vi "Extract BCD Parameter.vi"(8 "Signed?":bool, 9 "numberofBits":i32=19, 10 "startBit":i32=10, 11 "Word":bool[](array[boolean])=[FALSE, FALSE, FALSE, FALSE, FALSE, FALSE, FALSE, FALSE, FALSE, FALSE, FALSE, TRUE, TRUE, FALSE, FALSE, FALSE, FALSE, TRUE, TRUE, TRUE, TRUE, FALSE, TRUE, FALSE, TRUE, FALSE, FALSE, TRUE, FALSE, TRUE, TRUE, FALSE]) -> (3 "BCD Parameter":dbl=25786.0)   [LabVIEW 2019]
doc: "This VI decodes a BCD (signed or not) parameter.\nWhen it's a BCD signed parameter, it's considered negative when SSM bits are 11. For any other combination, we consider it to be positive."
panel:
  # "LSB"
  # "MSB"
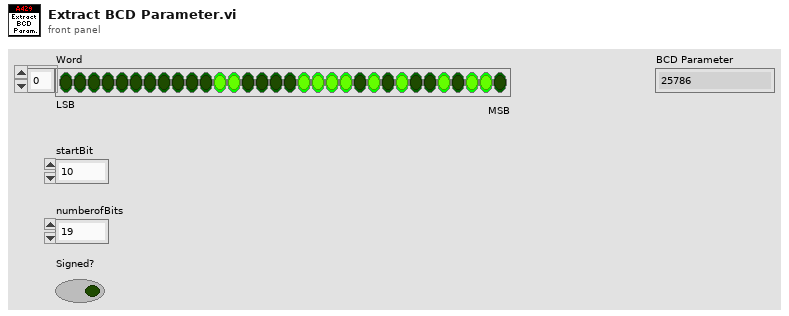
[diagram p1: front panel]
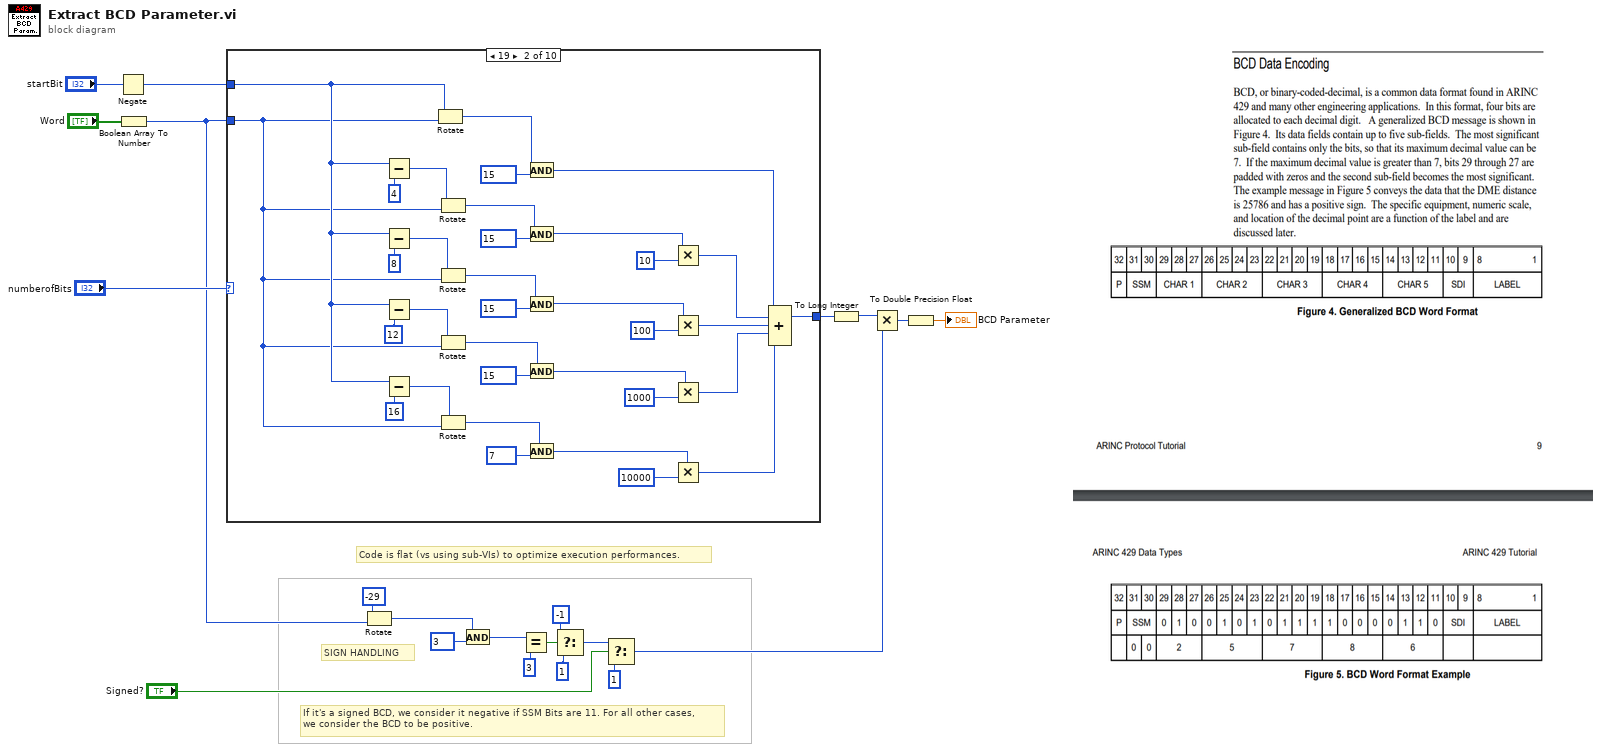
[diagram p0: block diagram]
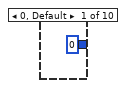
[diagram p2: hidden frame]
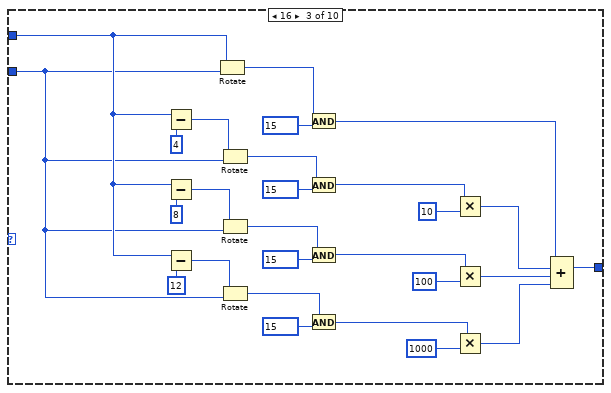
[diagram p3: hidden frame]
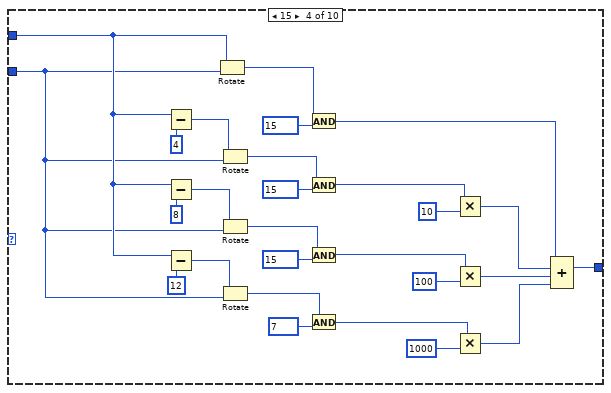
[diagram p4: hidden frame]
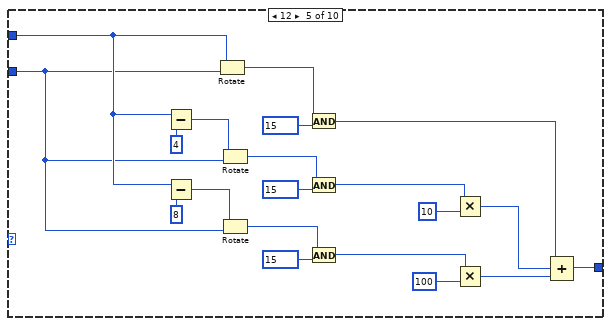
[diagram p5: hidden frame]
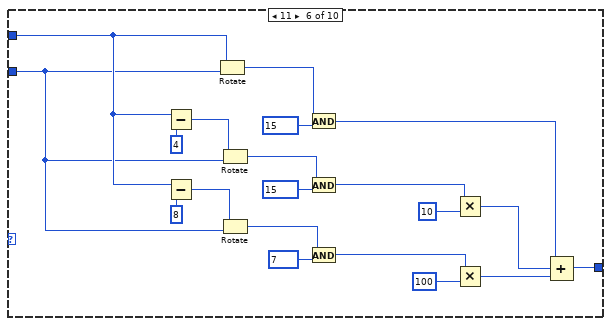
[diagram p6: hidden frame]
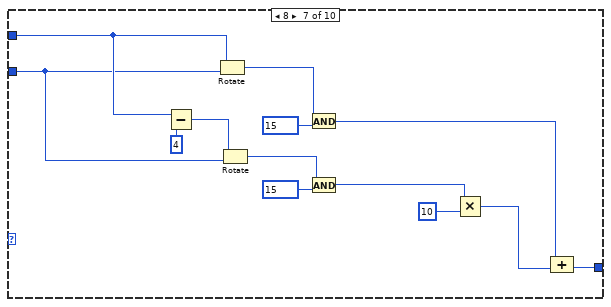
[diagram p7: hidden frame]
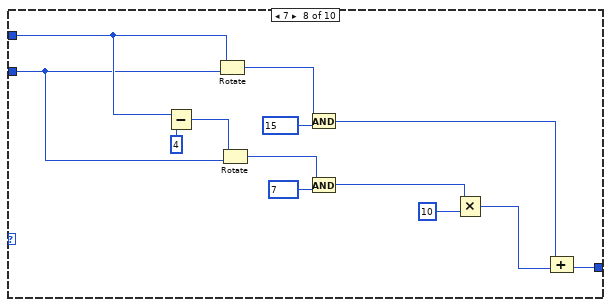
[diagram p8: hidden frame]
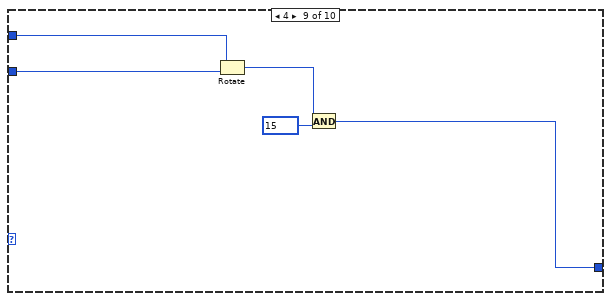
[diagram p9: hidden frame]
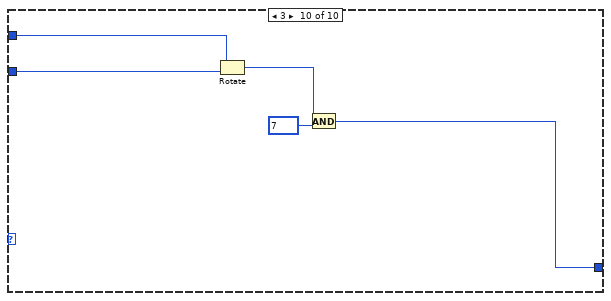
[diagram p10: hidden frame]
diagram:
  # "Code is flat (vs using sub-VIs) to optimize execution performances."
  # "If it's a signed BCD, we consider it negative if SSM Bits are 11. For all other cases,\nwe consider the BCD to be positive."
  # "SIGN HANDLING"
  n1 = Negate(x="startBit") -> (-x=w8:i32)
  n2 = Boolean Array To Number(Boolean array="Word") -> (number=w3:u32)
  n3 = case shown="19" "numberofBits" {
    tunnel: w8 -> [_ w25 w59 w86 w113 w133 w153 w166 w179 w184]
    tunnel: w3 -> [_ w24 w58 w85 w112 w132 w152 w165 w178 w183]
    tunnel: [u32 0 w23 w57 w84 w111 w131 w151 w164 w177 w182] -> w9
    frame 0, Default {
    }
    frame 19 {
      n4 = Subtract(x=w25, y=4) -> (x-y=w48:i32)
      n5 = Subtract(x=w25, y=8) -> (x-y=w42:i32)
      n6 = Subtract(x=w25, y=12) -> (x-y=w26:i32)
      n7 = Subtract(x=w25, y=16) -> (x-y=w27:i32)
      n8 = Rotate(1:w24, 2:w25) -> (0:w56:u32)
      n9 = Rotate(1:w24, 2:w48) -> (0:w52:u32)
      n10 = Rotate(1:w24, 2:w42) -> (0:w46:u32)
      n11 = Rotate(1:w24, 2:w26) -> (0:w40:u32)
      n12 = Rotate(1:w24, 2:w27) -> (0:w34:u32)
      n13 = And(x=w56, y=u32 15) -> (x .and. y?=w53:u32)
      n14 = And(x=w52, y=u32 15) -> (x .and. y?=w50:u32)
      n15 = And(x=w46, y=u32 15) -> (x .and. y?=w44:u32)
      n16 = And(x=w40, y=u32 15) -> (x .and. y?=w38:u32)
      n17 = And(x=w34, y=u32 7) -> (x .and. y?=w32:u32)
      n18 = Multiply(x=w50, y=u32 10) -> (x*y=w37:u32)
      n19 = Multiply(x=w44, y=u32 100) -> (x*y=w36:u32)
      n20 = Multiply(x=w38, y=u32 1000) -> (x*y=w31:u32)
      n21 = Multiply(x=w32, y=u32 10000) -> (x*y=w30:u32)
      n22 = Compound Arithmetic op=ADD(w53, w37, w36, w31, w30) -> (w23:u32)
    }
    frame 16 {
      n23 = Subtract(x=w59, y=4) -> (x-y=w75:i32)
      n24 = Subtract(x=w59, y=8) -> (x-y=w69:i32)
      n25 = Subtract(x=w59, y=12) -> (x-y=w60:i32)
      n26 = Rotate(1:w58, 2:w59) -> (0:w83:u32)
      n27 = Rotate(1:w58, 2:w75) -> (0:w79:u32)
      n28 = Rotate(1:w58, 2:w69) -> (0:w73:u32)
      n29 = Rotate(1:w58, 2:w60) -> (0:w67:u32)
      n30 = And(x=w83, y=u32 15) -> (x .and. y?=w80:u32)
      n31 = And(x=w79, y=u32 15) -> (x .and. y?=w77:u32)
      n32 = And(x=w73, y=u32 15) -> (x .and. y?=w71:u32)
      n33 = And(x=w67, y=u32 15) -> (x .and. y?=w65:u32)
      n34 = Multiply(x=w77, y=u32 10) -> (x*y=w64:u32)
      n35 = Multiply(x=w71, y=u32 100) -> (x*y=w63:u32)
      n36 = Multiply(x=w65, y=u32 1000) -> (x*y=w62:u32)
      n37 = Compound Arithmetic op=ADD(w80, w64, w63, w62) -> (w57:u32)
    }
    frame 15 {
      n38 = Subtract(x=w86, y=4) -> (x-y=w102:i32)
      n39 = Subtract(x=w86, y=8) -> (x-y=w96:i32)
      n40 = Subtract(x=w86, y=12) -> (x-y=w87:i32)
      n41 = Rotate(1:w85, 2:w86) -> (0:w110:u32)
      n42 = Rotate(1:w85, 2:w102) -> (0:w106:u32)
      n43 = Rotate(1:w85, 2:w96) -> (0:w100:u32)
      n44 = Rotate(1:w85, 2:w87) -> (0:w94:u32)
      n45 = And(x=w110, y=u32 15) -> (x .and. y?=w107:u32)
      n46 = And(x=w106, y=u32 15) -> (x .and. y?=w104:u32)
      n47 = And(x=w100, y=u32 15) -> (x .and. y?=w98:u32)
      n48 = And(x=w94, y=u32 7) -> (x .and. y?=w92:u32)
      n49 = Multiply(x=w104, y=u32 10) -> (x*y=w91:u32)
      n50 = Multiply(x=w98, y=u32 100) -> (x*y=w90:u32)
      n51 = Multiply(x=w92, y=u32 1000) -> (x*y=w89:u32)
      n52 = Compound Arithmetic op=ADD(w107, w91, w90, w89) -> (w84:u32)
    }
    frame 12 {
      n53 = Subtract(x=w113, y=4) -> (x-y=w122:i32)
      n54 = Subtract(x=w113, y=8) -> (x-y=w116:i32)
      n55 = Rotate(1:w112, 2:w113) -> (0:w130:u32)
      n56 = Rotate(1:w112, 2:w122) -> (0:w126:u32)
      n57 = Rotate(1:w112, 2:w116) -> (0:w120:u32)
      n58 = And(x=w130, y=u32 15) -> (x .and. y?=w127:u32)
      n59 = And(x=w126, y=u32 15) -> (x .and. y?=w124:u32)
      n60 = And(x=w120, y=u32 15) -> (x .and. y?=w118:u32)
      n61 = Multiply(x=w124, y=u32 10) -> (x*y=w115:u32)
      n62 = Multiply(x=w118, y=u32 100) -> (x*y=w114:u32)
      n63 = Compound Arithmetic op=ADD(w127, w115, w114) -> (w111:u32)
    }
    frame 11 {
      n64 = Subtract(x=w133, y=4) -> (x-y=w142:i32)
      n65 = Subtract(x=w133, y=8) -> (x-y=w136:i32)
      n66 = Rotate(1:w132, 2:w133) -> (0:w150:u32)
      n67 = Rotate(1:w132, 2:w142) -> (0:w146:u32)
      n68 = Rotate(1:w132, 2:w136) -> (0:w140:u32)
      n69 = And(x=w150, y=u32 15) -> (x .and. y?=w147:u32)
      n70 = And(x=w146, y=u32 15) -> (x .and. y?=w144:u32)
      n71 = And(x=w140, y=u32 7) -> (x .and. y?=w138:u32)
      n72 = Multiply(x=w144, y=u32 10) -> (x*y=w135:u32)
      n73 = Multiply(x=w138, y=u32 100) -> (x*y=w134:u32)
      n74 = Compound Arithmetic op=ADD(w147, w135, w134) -> (w131:u32)
    }
    frame 8 {
      n75 = Subtract(x=w153, y=4) -> (x-y=w155:i32)
      n76 = Rotate(1:w152, 2:w153) -> (0:w163:u32)
      n77 = Rotate(1:w152, 2:w155) -> (0:w159:u32)
      n78 = And(x=w163, y=u32 15) -> (x .and. y?=w160:u32)
      n79 = And(x=w159, y=u32 15) -> (x .and. y?=w157:u32)
      n80 = Multiply(x=w157, y=u32 10) -> (x*y=w154:u32)
      n81 = Compound Arithmetic op=ADD(w160, w154) -> (w151:u32)
    }
    frame 7 {
      n82 = Subtract(x=w166, y=4) -> (x-y=w168:i32)
      n83 = Rotate(1:w165, 2:w166) -> (0:w176:u32)
      n84 = Rotate(1:w165, 2:w168) -> (0:w172:u32)
      n85 = And(x=w176, y=u32 15) -> (x .and. y?=w173:u32)
      n86 = And(x=w172, y=u32 7) -> (x .and. y?=w170:u32)
      n87 = Multiply(x=w170, y=u32 10) -> (x*y=w167:u32)
      n88 = Compound Arithmetic op=ADD(w173, w167) -> (w164:u32)
    }
    frame 4 {
      n89 = Rotate(1:w178, 2:w179) -> (0:w181:u32)
      n90 = And(x=w181, y=u32 15) -> (x .and. y?=w177:u32)
    }
    frame 3 {
      n91 = Rotate(1:w183, 2:w184) -> (0:w186:u32)
      n92 = And(x=w186, y=u32 7) -> (x .and. y?=w182:u32)
    }
  }
  n93 = Rotate(1:w3, 2:-29 ("x")) -> (0:w5:u32)
  n94 = And(x=w5, y=u32 3) -> (x .and. y?=w4:u32)
  n95 = Equal?(x=w4, y=u32 3) -> (x = y?=w17:bool)
  n96 = Select(t=-1, s=w17, f=1 ("t")) -> (s? t:f=w14:i32)
  n97 = Select(t=w14, s="Signed?", f=1) -> (s? t:f=w6:i32)
  n98 = To Long Integer(number=w9) -> (32bit integer=w7:i32)
  n99 = Multiply(x=w7, y=w6) -> (x*y=w2:i32)
  n100 = To Double Precision Float(number=w2) -> (double precision float=→"BCD Parameter":dbl)
